vi "test-cubic-spline-00.vi"() -> ()   [LabVIEW 2019]
uses:
  <vilib>/Rock Robotics/WPI/ThirdParty/JAS_Junk/TrajLib/POSEwCURVATURE.ctl
  <vilib>/Rock Robotics/WPI/ThirdParty/JAS_Junk/TrajLib/POSE2D.ctl
  <vilib>/Rock Robotics/WPI/ThirdParty/JAS_Junk/TrajLib/TRANSLATION2D.ctl
  <vilib>/Rock Robotics/WPI/ThirdParty/JAS_Junk/TrajLib/ROTATION2D.ctl
  <vilib>/Rock Robotics/WPI/ThirdParty/JAS_Junk/TrajLib/Rotation_CreateAngle.vi
  <vilib>/Rock Robotics/WPI/ThirdParty/JAS_Junk/TrajLib/Translation_Create.vi
  <vilib>/Rock Robotics/WPI/ThirdParty/JAS_Junk/TrajLib/Util_CalcDist.vi
  <vilib>/Rock Robotics/WPI/ThirdParty/JAS_Junk/TrajLib/Trajectory_Library.lvlib
panel:
  out "All Interior \nwayPoints\nFound (True)":bool
  out "end rot = 0":dbl
  out "end y = 0":dbl
  out "end x = 0":dbl
  out "start rot = 0":dbl
  out "start y = 0":dbl
  out "start x = 0":dbl
  out "max dtheta < 0.0872":dbl
  out "max dy < 0.00127":dbl
  out "max dx  < 0.127":dbl
  out "Overall Error":errorcluster
  out "Elements":i32
  out "Create Spline Error":errorcluster
  out "SplinePoses\nWCurve":T1[](array[typedef]) {"POSE"."ROTATION"."SIN" format="%13.4f"; "POSE"."ROTATION"."COS" format="%13.4f"; "POSE"."ROTATION"."VALUE" format="%13.4f"; "POSE"."TRANSLATION"."Y" format="%14.3f"; "POSE"."TRANSLATION"."X" format="%14.3f"}
  out "Elapsed Time":dbl
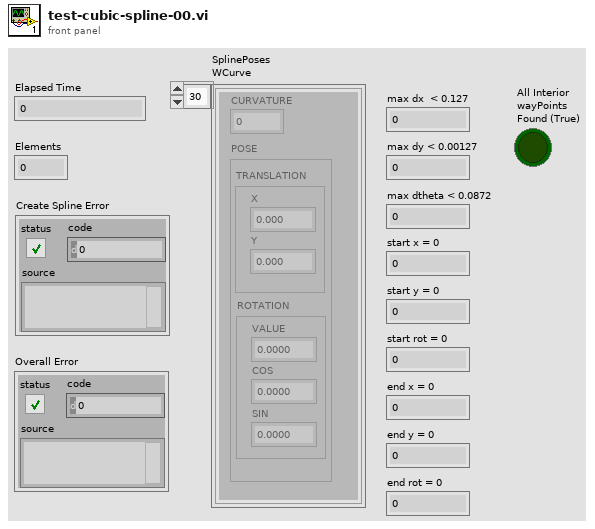
[diagram p1: front panel]
types:
  T1 = typedef "Trajectory_Library.lvlib/POSEwCURVATURE.ctl" = cluster{"CURVATURE":dbl, "POSE":T2}
  T2 = typedef "Trajectory_Library.lvlib/POSE2D.ctl" = cluster{"TRANSLATION":T3, "ROTATION":T4}
  T3 = typedef "Trajectory_Library.lvlib/TRANSLATION2D.ctl" = cluster{"X":dbl, "Y":dbl}
  T4 = typedef "Trajectory_Library.lvlib/ROTATION2D.ctl" = cluster{"VALUE":dbl, "COS":dbl, "SIN":dbl}
  T5 = typedef "Trajectory_Library.lvlib/SPLINE_CTRL_VECTOR.ctl" = cluster{"Xs":dbl[], "Ys":dbl[]}
  T6 = typedef "Trajectory_Library.lvlib/SPLINE.ctl" = cluster{"Degree":i32, "Coefficients":T7}
  T7 = typedef "NI_Matrix.lvlib/RealMatrix.ctl" = dbl[][]
  T8 = typedef "Trajectory_Library.lvlib/TWIST2D.ctl" = cluster{"dX":dbl, "dY":dbl, "dTHETA":dbl}
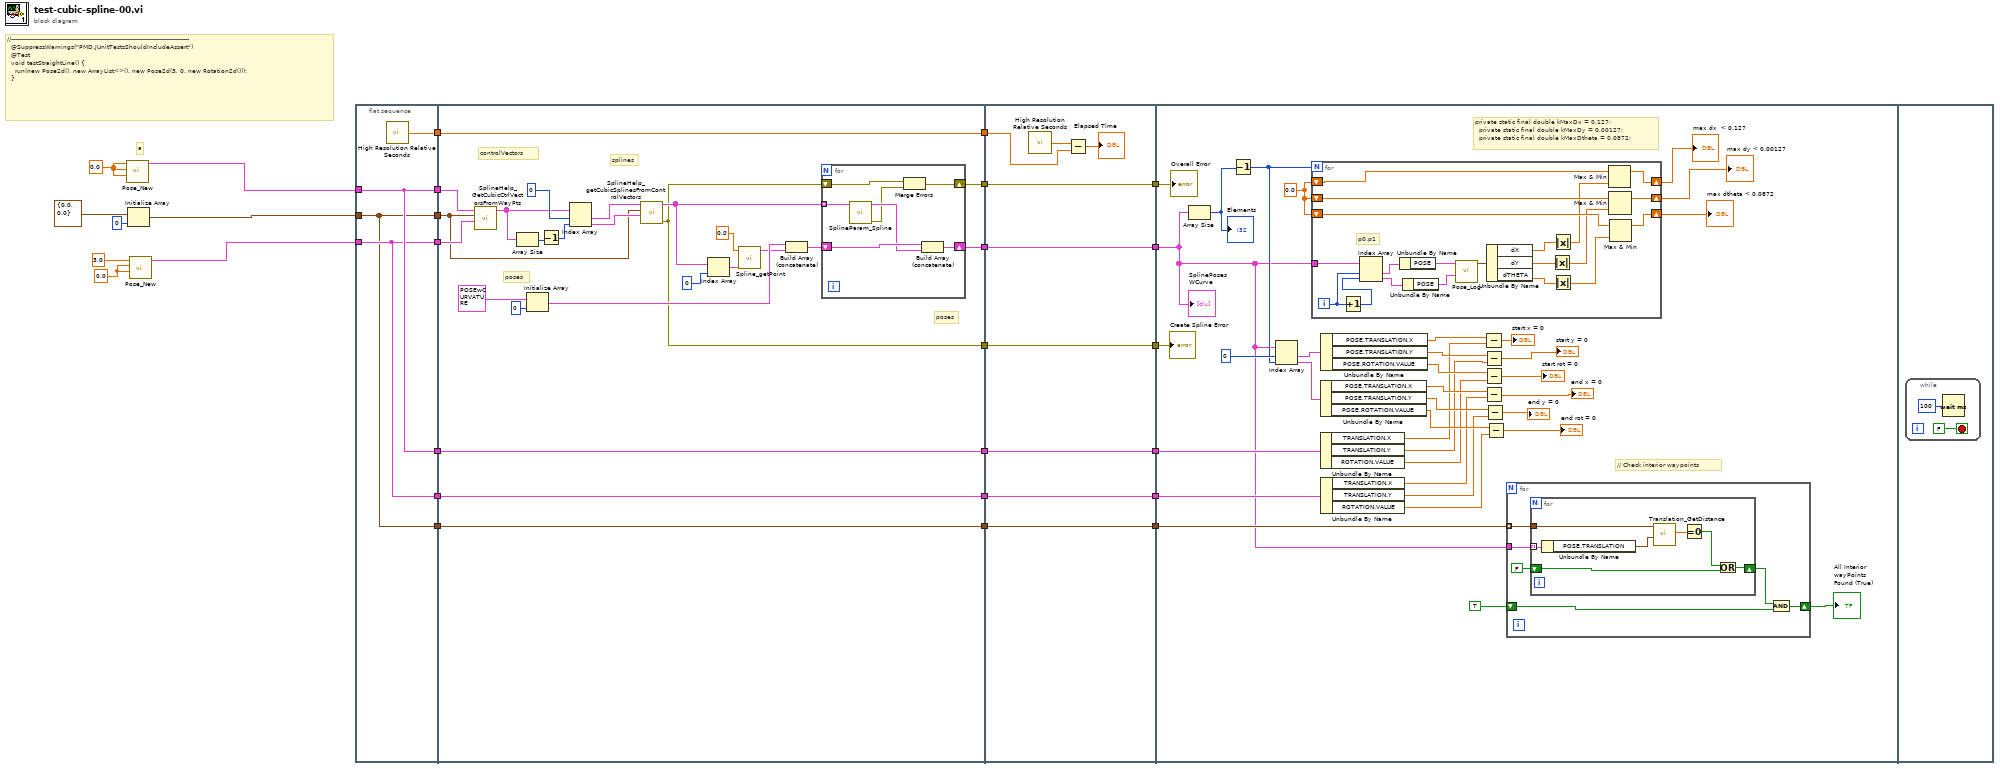
[diagram p0: block diagram]
diagram:
  w24 = 0.0 ("Y")
  w26 = 0.0 ("X")
  # "a"
  # "//-----------------------------------------------------------------------------------------\n  @SuppressWarnings(\"PMD.JUnitTestsShouldIncludeAssert\")\n  @Test\n  void testStraightLine() {\n    run(new Pose2d(), new ArrayList<>(), new Pose2d(3, 0, new Rotation2d()));\n  }"
  n1 = call <vilib>:"Pose_New.vi"("Heading"=w26, "Y"=w26, "X"=w26) -> ("out POSe"=w23:T2)  [unwired: 8 in]
  n2 = Initialize Array(T3 {"X"=0.0, "Y"=0.0} ("TRANSLATION"), 0 ("dimension size")) -> (w21:T3[])
  n3 = call <vilib>:"Pose_New.vi"("Heading"=w24, "Y"=w24, "X"=3.0) -> ("out POSe"=w19:T2)  [unwired: 8 in]
  n4 = flat-sequence {
    tunnel: w23 -> [w31]
    tunnel: [w31] -> w22
    tunnel: w21 -> [w29]
    tunnel: [w29] -> w20
    tunnel: w19 -> [w30]
    tunnel: [w30] -> w18
    tunnel: [w32] -> w17
    tunnel: [w31] -> w9
    tunnel: [w30] -> w6
    tunnel: [w29] -> w1
    tunnel: w22 -> [w57]
    tunnel: w20 -> [w49]
    tunnel: w18 -> [w56]
    tunnel: [w48] -> w16
    tunnel: w17 -> [w48]
    tunnel: [w38] -> w15
    tunnel: [w37] -> w13
    tunnel: [w36] -> w11
    tunnel: w9 -> [w35]
    tunnel: [w35] -> w8
    tunnel: w6 -> [w34]
    tunnel: [w34] -> w5
    tunnel: [w33] -> w2
    tunnel: w1 -> [w33]
    tunnel: w16 -> [w73]
    tunnel: w15 -> [w72]
    tunnel: [w72] -> w14
    tunnel: w13 -> [w71]
    tunnel: [w71] -> w12
    tunnel: w11 -> [w70]
    tunnel: [w70] -> w10
    tunnel: w8 -> [w67]
    tunnel: [w67] -> w7
    tunnel: w5 -> [w66]
    tunnel: [w66] -> w4
    tunnel: [w65] -> w3
    tunnel: w2 -> [w65]
    tunnel: w14 -> [w76]
    tunnel: w12 -> [w108]
    tunnel: w10 -> [w107]
    tunnel: w7 -> [w101]
    tunnel: w4 -> [w100]
    tunnel: w3 -> [w77]
    frame #0 {
      n5 = call <vilib>:"High Resolution Relative Seconds.vi"() -> ("relative seconds"=w32:dbl)
    }
    frame #1 {
      # "poses"
      # "poses"
      # "splines"
      # "controlVectors"
      n6 = call <vilib>:"SplineHelp_GetCubicCtrlVectorsFromWayPts.vi"("Enging POSE"=w56, "Interior WAYPOINTS"=w49, "Starting POSE"=w57) -> ("SplineControlVectors"=w53:T5[])  [unwired: 8 in]
      n7 = Array Size(array=w53) -> (size(s)=w54:i32)
      n8 = Initialize Array(T1 {"CURVATURE"=0.0, "POSE"={"TRANSLATION"={"X"=0.0, "Y"=0.0}, "ROTATION"={"VALUE"=0.0, "COS"=1.0, "SIN"=0.0}}} ("POSEwCURVATURE"), 0 ("dimension size")) -> (w42:T1[])
      n9 = Decrement(x=w54) -> (x-1=w52:i32)
      n10 = Index Array(array=w53, index #1=0 ("index"), index #2=w52) -> (element #1=w51:T5, element #2=w50:T5)
      n11 = call <vilib>:"SplineHelp_getCubicSplinesFromControlVectors.vi"("endCtrlVector"=w50, "InternalWaypoints"=w49, "startCtrlVector"=w51) -> ("error out"=w37:errorcluster, "splines"=w39:T6[])  [unwired: 3 in, 4 out]
      n12 = Index Array(array=w39, index=0) -> (element=w44:T6)
      n13 = call <vilib>:"Spline_getPoint.vi"("inputSPLINE"=w44, "Time"=0.0) -> ("POSEwCURVATURE"=w41:T1)  [unwired: 9 in]
      n14 = Build Array (concatenate)(w42, w41) -> (w40:T1[])
      n15 = for {
        shift-right: [w61] -> w38
        shift-left: w40 -> [w63]
        tunnel: w39 -> [w64] mode=indexing
        shift-right: [w59] -> w36
        shift-left: w37 -> [w60]
        n16 = call <vilib>:"SplineParam_Spline.vi"("inputSPLINE"=w64) -> ("error out"=w58:errorcluster, "outputPOSEwCURVATURE"=w62:T1[])  [unwired: 9 in]
        n17 = Merge Errors(w60, w58) -> (w59:errorcluster)
        n18 = Build Array (concatenate)(w63, w62) -> (w61:T1[])
      }
    }
    frame #2 {
      n19 = call <vilib>:"High Resolution Relative Seconds.vi"() -> ("relative seconds"=w68:dbl)
      n20 = Subtract(x=w68, y=w73) -> (x-y=→"Elapsed Time":dbl)
    }
    frame #3 {
      w105 = 0.0
      # "// Check interior waypoints"
      # "private static final double kMaxDx = 0.127;\n  private static final double kMaxDy = 0.00127;\n  private static final double kMaxDtheta = 0.0872;"
      n21 = Array Size(array=w76) -> (size(s)=w106:i32)
      "Elements" <- w106
      n22 = Decrement(x=w106) -> (x-1=w98:i32)
      n23 = Index Array(array=w76, index #1=0 ("index"), index #2=w98) -> (element #1=w97:T1, element #2=w96:T1)
      n24 = for {
        N: w98 -> [_]
        tunnel: w76 -> [w139]
        shift-right: [w130] -> w104
        shift-left: w105 -> [w127]
        shift-right: [w128] -> w102
        shift-left: w105 -> [w125]
        shift-right: [w129] -> w103
        shift-left: w105 -> [w126]
        i -> [w141]
        # "p0,p1"
        n25 = Increment(x=w141) -> (x+1=w140:i32)
        n26 = Index Array(array=w139, index #1=w141, index #2=w140) -> (element #1=w138:T1, element #2=w137:T1)
        n27 = Unbundle By Name(w138) -> ("POSE"=w136:T2)
        n28 = Unbundle By Name(w137) -> ("POSE"=w135:T2)
        n29 = call <vilib>:"Pose_Log.vi"("end POSE"=w135, "in POSE"=w136) -> ("out TWIST"=w134:T8)  [unwired: 9 in]
        n30 = Unbundle By Name(w134) -> ("dX"=w131:dbl, "dY"=w132:dbl, "dTHETA"=w133:dbl)
        n31 = Absolute Value(x=w132) -> (abs(x)=w123:dbl)
        n32 = Absolute Value(x=w131) -> (abs(x)=w124:dbl)
        n33 = Absolute Value(x=w133) -> (abs(x)=w122:dbl)
        n34 = Max & Min(x=w127, y=w124) -> (max(x,y)=w130:dbl)  [unwired: 1 out]
        n35 = Max & Min(x=w126, y=w123) -> (max(x,y)=w129:dbl)  [unwired: 1 out]
        n36 = Max & Min(x=w125, y=w122) -> (max(x,y)=w128:dbl)  [unwired: 1 out]
      }
      "max dx  < 0.127" <- w104
      "max dy < 0.00127" <- w103
      "max dtheta < 0.0872" <- w102
      n37 = Unbundle By Name(w96) -> ("POSE.TRANSLATION.X"=w92:dbl, "POSE.TRANSLATION.Y"=w91:dbl, "POSE.ROTATION.VALUE"=w90:dbl)
      n38 = Unbundle By Name(w101) -> ("TRANSLATION.X"=w89:dbl, "TRANSLATION.Y"=w88:dbl, "ROTATION.VALUE"=w87:dbl)
      n39 = Unbundle By Name(w97) -> ("POSE.TRANSLATION.X"=w95:dbl, "POSE.TRANSLATION.Y"=w94:dbl, "POSE.ROTATION.VALUE"=w93:dbl)
      n40 = Unbundle By Name(w100) -> ("TRANSLATION.X"=w86:dbl, "TRANSLATION.Y"=w85:dbl, "ROTATION.VALUE"=w84:dbl)
      n41 = Subtract(x=w95, y=w89) -> (x-y=→"start x = 0":dbl)
      n42 = Subtract(x=w94, y=w88) -> (x-y=→"start y = 0":dbl)
      n43 = Subtract(x=w93, y=w87) -> (x-y=→"start rot = 0":dbl)
      n44 = Subtract(x=w92, y=w86) -> (x-y=→"end x = 0":dbl)
      n45 = Subtract(x=w91, y=w85) -> (x-y=→"end y = 0":dbl)
      n46 = Subtract(x=w90, y=w84) -> (x-y=→"end rot = 0":dbl)
      n47 = for {
        tunnel: w77 -> [w109] mode=indexing
        tunnel: w76 -> [w114]
        shift-right: [w113] -> w74
        shift-left: TRUE -> [w112]
        n48 = for {
          tunnel: w114 -> [w118] mode=indexing
          shift-right: [w121] -> w110
          shift-left: FALSE -> [w120]
          tunnel: w109 -> [w119]
          n49 = Unbundle By Name(w118) -> ("POSE.TRANSLATION"=w117:T3)
          n50 = call <vilib>:"Translation_GetDistance.vi"("other Translation"=w117, "In Translation"=w119) -> ("Distance"=w116:dbl)  [unwired: 9 in]
          n51 = Equal To 0?(x=w116) -> (x = 0?=w115:bool)
          n52 = Or(x=w115, y=w120) -> (x .or. y?=w121:bool)
        }
        n53 = And(x=w110, y=w112) -> (x .and. y?=w113:bool)
      }
      "All Interior \nwayPoints\nFound (True)" <- w74
      "SplinePoses\nWCurve" <- w76
      "Create Spline Error" <- w108
      "Overall Error" <- w107
    }
    frame #4 {
      n54 = while {
        stop <- FALSE stop-if-true
        n55 = Wait (ms)(milliseconds to wait=u32 100) -> ()  [unwired: 1 out]
      }
    }
  }
